vi "UndoTurns.vi"(2 "MoveComplete?":refnum<vi>, 3 "#Turns":refnum<vi>, 4 "error in (no error)":errorcluster, 5 "MG17Motor":refnum<k7>(container)) -> (0 "error out":errorcluster, 1 "MG17MotorOut":refnum<k7>)   [LabVIEW 2010]
panel:
  out "CurrentStepSize":dbl
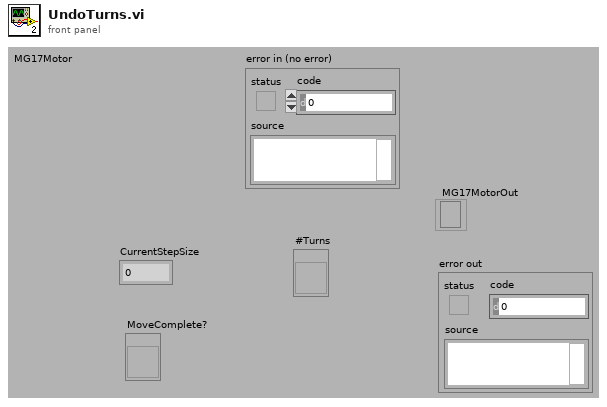
[diagram p1: front panel]
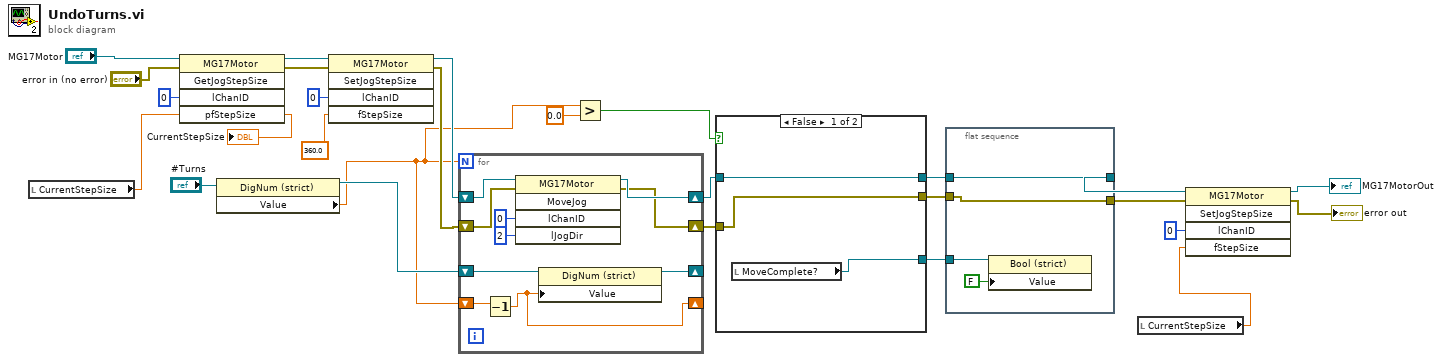
[diagram p0: block diagram]
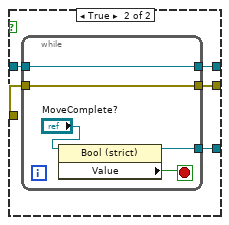
[diagram p2: hidden frame]
diagram:
  n1 = local read "CurrentStepSize"() -> (w25:dbl)
  n2 = invoke class="MG17Motor" method="GetJogStepSize"(reference="MG17Motor", error in="error in (no error)", "lChanID"=0, "pfStepSize"=w25) -> (reference out=w22:refnum<k7>, error out=w21:errorcluster, "pfStepSize"=→"CurrentStepSize":sgl)  [unwired: 1 in, 2 out]
  n3 = property class="DigNum (strict)"(reference="#Turns") -> (reference out=w15:refnum<vi>, "Value"=w3:dbl)  [unwired: 1 in, 1 out]
  n4 = invoke class="MG17Motor" method="SetJogStepSize"(reference=w22, error in=w21, "lChanID"=0, "fStepSize"=sgl 360.0) -> (reference out=w17:refnum<k7>, error out=w18:errorcluster)  [unwired: 1 in, 3 out]
  n5 = for {
    N: w3 -> [_]
    shift-right: [w33] -> w10
    shift-left: w17 -> [w35]
    shift-right: [w32] -> w9
    shift-left: w18 -> [w34]
    shift-right: [w30] -> _
    shift-left: w15 -> [w31]
    shift-right: [w28] -> _
    shift-left: w3 -> [w29]
    n6 = Decrement(x=w29) -> (x-1=w28:dbl)
    n7 = invoke class="MG17Motor" method="MoveJog"(reference=w35, error in=w34, "lChanID"=0, "lJogDir"=2) -> (reference out=w33:refnum<k7>, error out=w32:errorcluster)  [unwired: 1 in, 3 out]
    n8 = property class="DigNum (strict)"(reference=w31, "Value"=w28) -> (reference out=w30:refnum<vi>)  [unwired: 1 in, 1 out]
  }
  n9 = Greater?(x=w3, y=0.0) -> (0:w1:bool)
  n10 = case shown="False" w1 {
    tunnel: w10 -> [w40 w45]
    tunnel: w9 -> [w39 w44]
    tunnel: [w40 w43] -> w8
    tunnel: [w39 w42] -> w6
    tunnel: [w38 w41] -> w4
    frame False {
      n11 = local read "MoveComplete?"() -> (w38:refnum<vi>)
    }
    frame True {
      n12 = while {
        tunnel: w45 -> [w49]
        tunnel: w44 -> [w50]
        tunnel: [w50] -> w42
        tunnel: [w49] -> w43
        tunnel: [w46] -> w41
        stop <- w47 stop-if-true
        n13 = property class="Bool (strict)"(reference="MoveComplete?") -> (reference out=w46:refnum<vi>, "Value"=w47:bool)  [unwired: 1 in, 1 out]
      }
    }
  }
  n14 = flat-sequence {
    tunnel: w8 -> [w54]
    tunnel: [w54] -> w7
    tunnel: w6 -> [w53]
    tunnel: [w53] -> w5
    tunnel: w4 -> [w52]
    frame #0 {
      n15 = property class="Bool (strict)"(reference=w52, "Value"=FALSE) -> ()  [unwired: 1 in, 2 out]
    }
  }
  n16 = local read "CurrentStepSize"() -> (w14:dbl)
  n17 = invoke class="MG17Motor" method="SetJogStepSize"(reference=w7, error in=w5, "lChanID"=0, "fStepSize"=w14) -> (reference out=→"MG17MotorOut":refnum<k7>, error out=→"error out":errorcluster)  [unwired: 1 in, 3 out]
